vi "AI Voltage Single Channel Measurement_Debug.vi"(6 "Measurement Mode":T2(ring)=enum."Single Channel : Multiple Samples", 8 "error in (no error)":errorcluster, 9 "Timing Settings":T1={"Sample Rate"=1000.0, "Number of Samples"=100}, 10 "Channel Settings":T3={"Min Value"=-5.0, "Max Value"=5.0, "Terminal Configuration"=-1} {"Terminal Configuration" items=["default"=-1, "RSE"=10083, "NRSE"=10078, "Differential"=10106, "Pseudodifferential"=12529]}, 11 "Physical Channel":tag="Dev1/ai0") -> (0 "error out":errorcluster, 1 "Frequency":dbl=1000.0 format="%0.2f", 2 "Waveform Graph":waveform(dbl)(graph))   [LabVIEW 2022 SP3]
uses:
  Type Definitions/AI Channel Settings.ctl
  Type Definitions/Timing Settings.ctl
  niMIO.lvclass
  <vilib>/DAQmx/read.llb/DAQmx Read (Analog Wfm 1Chan NSamp).vi
  <vilib>/DAQmx/create/channels.llb/DAQmx Create Channel (AI-Voltage-Basic).vi
  <vilib>/DAQmx/configure/timing.llb/DAQmx Timing (Sample Clock).vi
  <vilib>/DAQmx/miscellaneous.llb/DAQmx Fill In Error Info.vi
  <vilib>/measure/matone.llb/Extract Single Tone Information 1 Chan.vi
  <vilib>/measure/mascope.llb/Pulse Measurements 1 chan.vi
  <resource>/objmgr/daqmx.rc
  <vilib>/measure/NI_MAPro.lvlib
panel:
  out "detected frequency":dbl format="%.2p"
  out "F-format string":string
  out "Array":dbl[](array[numeric])
  out "Waveform Graph 2":waveform(dbl)(graph)
  out "niMIO out":refnum<class "niMIO.lvclass">
  in  "niMIO in":refnum<class "niMIO.lvclass">
  out "Actual Sample Rate":dbl=1000.0 format="%0.2f"
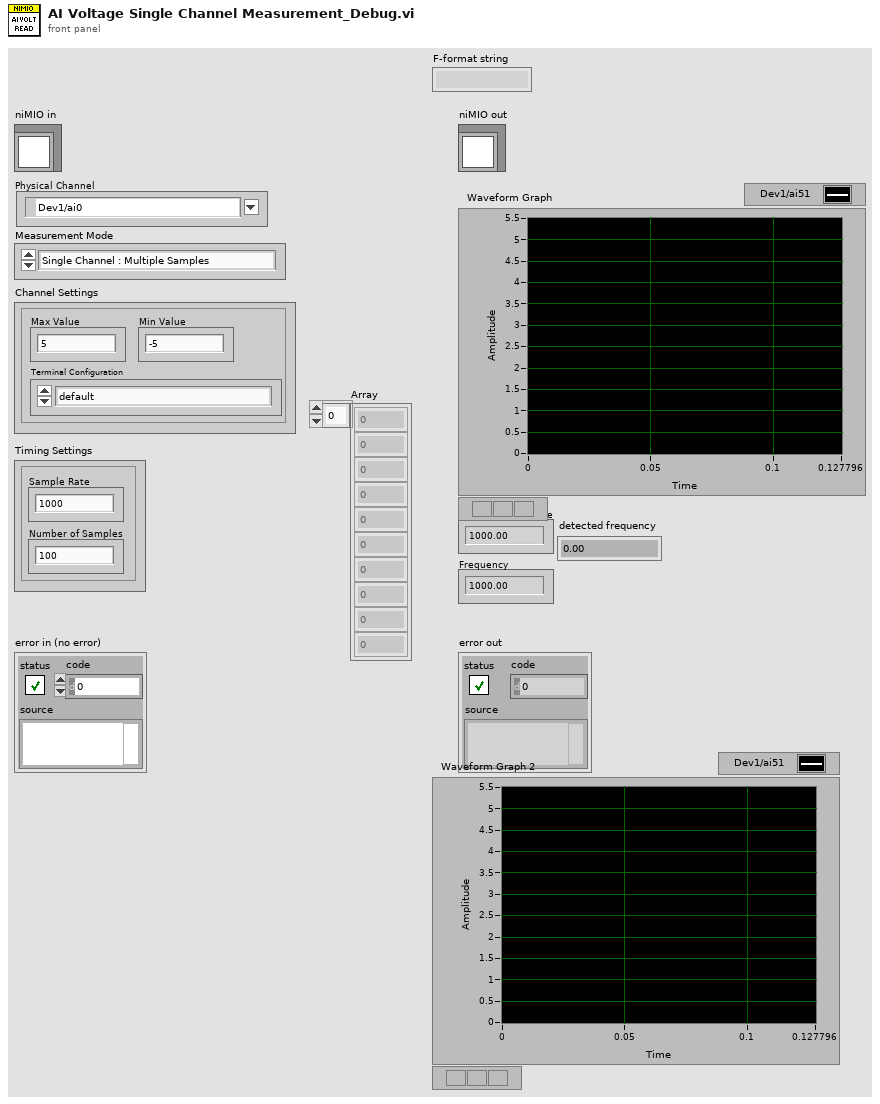
[diagram p1: front panel]
types:
  T1 = typedef "niMIO.lvclass/Timing Settings.ctl" = cluster{"Sample Rate":dbl, "Number of Samples":i32}
  T2 = enum16{"Single Channel : Single Sample", "Single Channel : Multiple Samples"}
  T3 = typedef "niMIO.lvclass/AI Channel Settings.ctl" = cluster{"Min Value":dbl, "Max Value":dbl, "Terminal Configuration":i32}
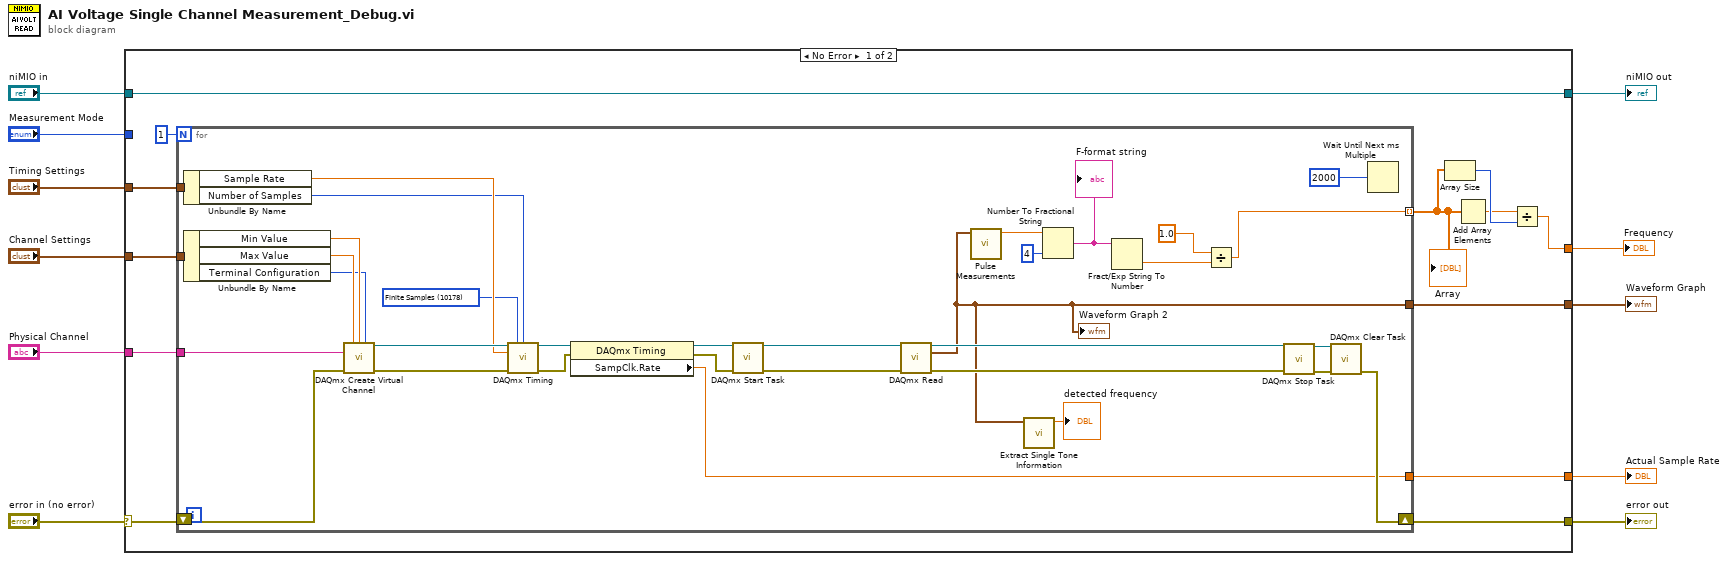
[diagram p0: block diagram]
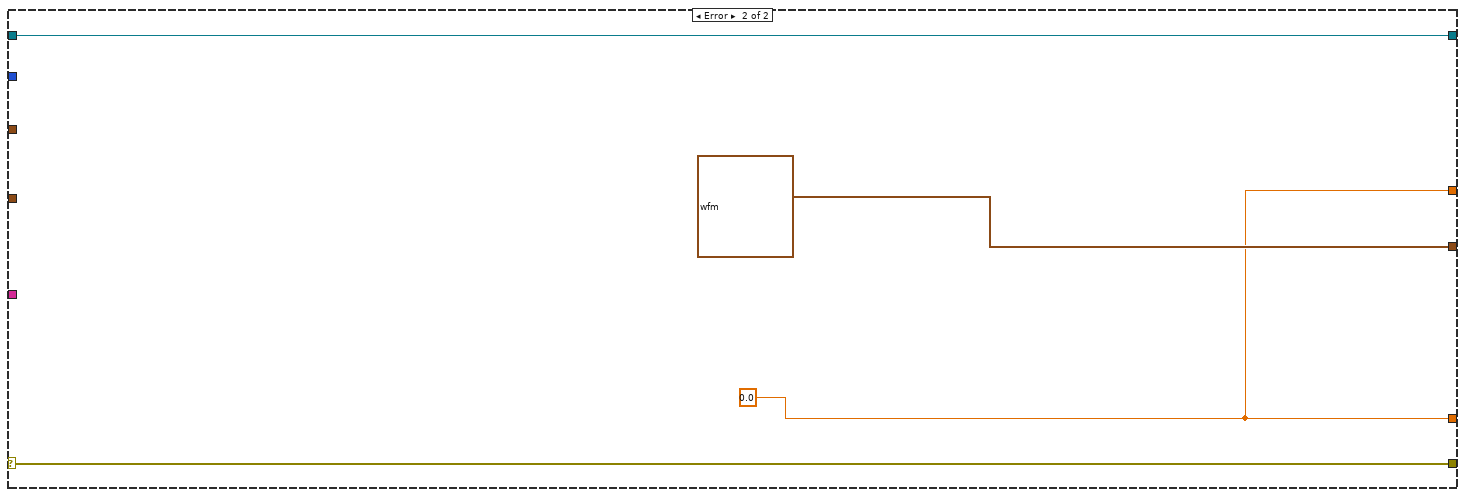
[diagram p2: hidden frame]
diagram:
  n1 = case shown="No Error" "error in (no error)" {
    selector: "error in (no error)" -> [w21 w61]
    tunnel: [w23 w61] -> w10
    tunnel: [w24 w60] -> w2
    tunnel: "niMIO in" -> [w24 w60]
    tunnel: "Channel Settings" -> [w22 _]
    tunnel: "Timing Settings" -> [w20 _]
    tunnel: [w19 w58] -> w9
    tunnel: "Measurement Mode" -> [_ _]
    tunnel: [w18 waveform(dbl) {"t0"=timestamp(0 s since 1904-01-01), "dt"=1.0, "Y"=[]} ("data")] -> w6
    tunnel: "Physical Channel" -> [w17 _]
    tunnel: [w13 w58] -> w1
    frame No Error {
      n2 = for {
        N: 1 -> [_]
        tunnel: w22 -> [w49]
        tunnel: w20 -> [w45]
        tunnel: [w38] -> w19
        tunnel: [w26] -> w18
        tunnel: w17 -> [w36]
        shift-right: [w56] -> w23
        shift-left: w21 -> [w46]
        tunnel: [w33] -> w12 mode=indexing
        w43 = 10178 items=["Finite Samples"=10178, "Continuous Samples"=10123, "Hardware Timed Single Point"=12522] ("sample mode")
        n3 = Unbundle By Name(w45) -> ("Sample Rate"=w44:dbl, "Number of Samples"=w37:i32)
        n4 = Unbundle By Name(w49) -> ("Min Value"=w48:dbl, "Max Value"=w47:dbl, "Terminal Configuration"=w35:i32)
        n5 = call-poly <vilib>:"DAQmx Create Virtual Channel.vi"("maximum value"=w47, "minimum value"=w48, "input terminal configuration"=w35, "physical channels"=w36, "error in"=w46) -> ("task out"=w51:refnum<k21>, "error out"=w55:errorcluster)  [unwired: 9 in]
        n6 = call-poly <vilib>:"DAQmx Timing.vi"("task/channels in"=w51, "sample mode"=w43, "samples per channel"=w37, "rate"=w44, "error in"=w55) -> ("task out"=w40:refnum<k21>, "error out"=w41:errorcluster)  [unwired: 9 in]
        n7 = property class="DAQmx Timing"(reference=w40, error in=w41) -> (reference out=w39:refnum<k21>, error out=w42:errorcluster, "SampClk.Rate"=w38:dbl)
        n8 = call <vilib>:"DAQmx Start Task.vi"("task/channels in"=w39, "error in"=w42) -> ("task out"=w50:refnum<k21>, "error out"=w34:errorcluster)  [unwired: 12 in]
        n9 = call-poly <vilib>:"DAQmx Read.vi"("task/channels in"=w50, "error in"=w34) -> ("task out"=w53:refnum<k21>, "data"=w26:waveform(dbl), "error out"=w54:errorcluster)  [unwired: 11 in]
        "Waveform Graph 2" <- w26
        n10 = call-poly <vilib>:"Pulse Measurements.vi"("signal in"=w26) -> ("period"=w30:dbl)  [unwired: 6 in, 4 out]
        n11 = call-poly <vilib>:"Extract Single Tone Information.vi"("time signal in"=w26) -> ("detected frequency"=→"detected frequency":dbl)  [unwired: 5 in, 5 out]
        n12 = Number To Fractional String(number=w30, precision (6)=i16 4) -> (F-format string=w31:string)  [unwired: 2 in]
        "F-format string" <- w31
        n13 = Fract/Exp String To Number(string=w31) -> (number=w29:dbl)  [unwired: 3 in, 1 out]
        n14 = Divide(x=1.0, y=w29) -> (x/y=w33:dbl)
        n15 = call <vilib>:"DAQmx Stop Task.vi"("task/channels in"=w53, "error in"=w54) -> ("task out"=w52:refnum<k21>, "error out"=w57:errorcluster)  [unwired: 12 in]
        n16 = call <vilib>:"DAQmx Clear Task.vi"("task in"=w52, "error in"=w57) -> ("error out"=w56:errorcluster)  [unwired: 13 in]
        n17 = Wait Until Next ms Multiple(millisecond multiple=u32 2000) -> ()  [unwired: 1 out]
      }
      "Array" <- w12
      n18 = Array Size(array=w12) -> (size(s)=w15:i32)
      n19 = Add Array Elements(numeric array=w12) -> (sum=w14:dbl)
      n20 = Divide(x=w14, y=w15) -> (x/y=w13:dbl)
    }
    frame Error {
      w58 = 0.0 ("SampClk.Rate")
    }
  }
  "error out" <- w10
  "Actual Sample Rate" <- w9
  "Waveform Graph" <- w6
  "niMIO out" <- w2
  "Frequency" <- w1
